vi "DIAdem Text Split.vi"(4 "error in (no error)":errorcluster, 6 "Number of Characters":i32, 7 "Full Input Text":string) -> (0 "error out":errorcluster, 3 "Output Strings":string[](array[string]))   [LabVIEW 2020]
doc: "Splits a text into an array of strings"
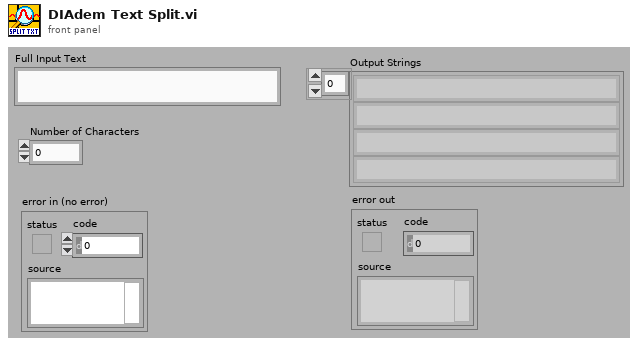
[diagram p1: front panel]
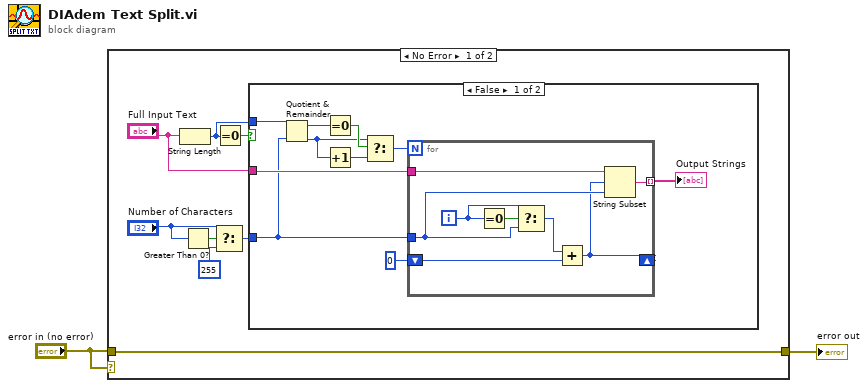
[diagram p0: block diagram]
diagram:
  n1 = case shown="No Error" "error in (no error)" {
    tunnel: [w7 w29] -> w1
    tunnel: "error in (no error)" -> [w7 w29]
    frame No Error {
      n2 = String Length(string="Full Input Text") -> (length=w8:i32)
      n3 = Greater Than 0?(x="Number of Characters") -> (x > 0?=w6:bool)
      n4 = Select(t="Number of Characters", s=w6, f=255) -> (s? t:f=w4:i32)
      n5 = Equal To 0?(x=w8) -> (x = 0?=w10:bool)
      n6 = case shown="False" w10 {
        tunnel: "Full Input Text" -> [w13 _]
        tunnel: w8 -> [w11 _]
        tunnel: w4 -> [w12 _]
        frame False {
          n7 = Quotient & Remainder(x=w11, y=w12) -> (x-y*floor(x/y)=w15:i32, floor(x/y)=w17:i32)
          n8 = Equal To 0?(x=w15) -> (x = 0?=w19:bool)
          n9 = Increment(x=w17) -> (x+1=w16:i32)
          n10 = Select(t=w17, s=w19, f=w16) -> (s? t:f=w18:i32)
          n11 = for {
            N: w18 -> [_]
            tunnel: [w23] -> w20 mode=indexing
            tunnel: w13 -> [w28]
            shift-right: [w24] -> _
            shift-left: 0 -> [w27]
            tunnel: w12 -> [w25]
            i -> [w22]
            n12 = Equal To 0?(x=w22) -> (x = 0?=w26:bool)
            n13 = Select(t=w22, s=w26, f=w25) -> (s? t:f=w21:i32)
            n14 = Add(x=w21, y=w27) -> (x+y=w24:i32)
            n15 = String Subset(string=w28, offset (0)=w24, length (rest)=w25) -> (substring=w23:string)
          }
          "Output Strings" <- w20
        }
        frame True {
        }
      }
    }
    frame Error {
    }
  }
  "error out" <- w1
